vi "Send StopHandler Event.vi"(8 "error in (no error)":errorcluster, 10 "Stop data":variant, 11 "Editor Handler in":refnum<class "Image Editor Handler.lvclass">) -> (0 "error out":errorcluster, 3 "Editor Handler out":refnum<class "Image Editor Handler.lvclass">)   [LabVIEW 2017, in "LV Image Editor Framework.lvlib" / "Image Editor Handler.lvclass"]
uses:
  Image Editor Handler.lvclass
  Image Editor Handler.lvclass/Image Editor Handler.ctl
  <vilib>/Utility/error.llb/Error Cluster From Error Code.vi
  <vilib>/ErrorRing/Error Ring.xnode
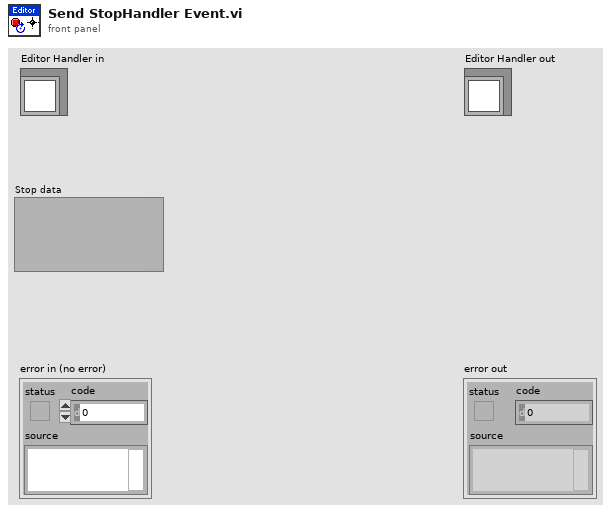
[diagram p1: front panel]
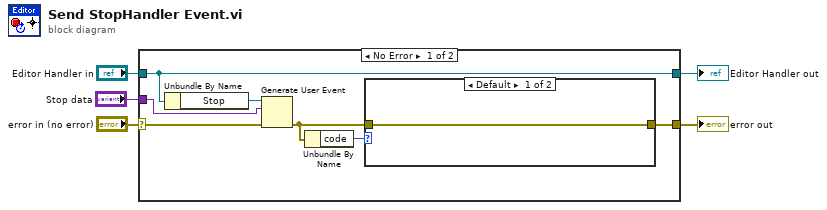
[diagram p0: block diagram]
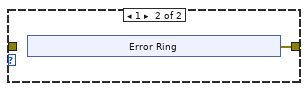
[diagram p2: hidden frame]
diagram:
  n1 = case shown="No Error" "error in (no error)" {
    selector: "error in (no error)" -> [w10 w21]
    tunnel: [w7 w21] -> w4
    tunnel: [w11 w20] -> w2
    tunnel: "Editor Handler in" -> [w11 w20]
    tunnel: "Stop data" -> [w9 _]
    frame No Error {
      n2 = Unbundle By Name(w11) -> ("Stop"=w12:refnum<user-event>)
      n3 = Generate User Event(user event=w12, event data cluster=w9, error in=w10) -> (error out=w6:errorcluster)  [unwired: 1 in, 1 out]
      n4 = Unbundle By Name(w6) -> ("code"=w8:i32)
      n5 = case shown="Default" w8 {
        tunnel: [w13 w14] -> w7
        tunnel: w6 -> [w13 _]
        frame Default {
        }
        frame 1 {
          n6 = xnode "Error Ring"() -> ("error out"=w14:errorcluster)
        }
      }
    }
    frame Error {
    }
  }
  "error out" <- w4
  "Editor Handler out" <- w2
